vi "control scan.vi"(6 "B scan number":i32, 7 "Stop":bool, 9 "Scan index":i32, 10 "Scan modes":T1(ring), 11 "External trigger":bool) -> (2 "Stop main":bool, 3 "Stop scan":bool)   [LabVIEW 2014]
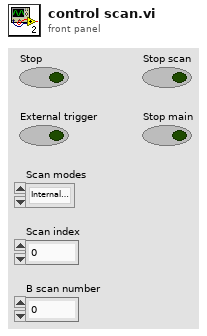
[diagram p1: front panel]
types:
  T1 = enum32{"Internal trigger", "External trigger", "Frequency Spectrum"}
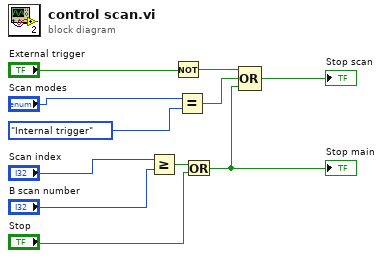
[diagram p0: block diagram]
diagram:
  n1 = Greater Or Equal?(x="Scan index", y="B scan number") -> (x >= y?=w5:bool)
  n2 = Not(x="External trigger") -> (.not. x?=w10:bool)
  n3 = Equal?(x="Scan modes", y=enum32{"Internal trigger", "External trigger"}."Internal trigger") -> (x = y?=w7:bool)
  n4 = Or(x=w5, y="Stop") -> (x .or. y?=w8:bool)
  "Stop main" <- w8
  n5 = Compound Arithmetic op=OR(w10, w7, w8) -> (→"Stop scan":bool)
